vi "Insert Into Array.vi"   [LabVIEW 2017, in "LVJSON.lvlib" / "JSON Array.lvclass"]
uses:
  JSON Array.lvclass
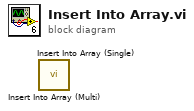
[diagram p0: block diagram]
diagram:
  n1 = call "Insert Into Array (Multi).vi"() -> ()  [unwired: 10 in, 2 out]
  n2 = call "Insert Into Array (Single).vi"() -> ()  [unwired: 10 in, 2 out]
